vi "MU Calibration Get Analyze Result Log.vi"(8 "error in (no error)":errorcluster, 9 "logLevel":u32, 10 "logDestSize":u64=1024, 11 "analyzeResult":T1) -> (0 "error out (no error)":errorcluster, 2 "logDest":string, 3 "size":u64=1024)   [LabVIEW 2017, in "MU_3SL_interface.lvlib"]
uses:
  MU_3SL_interface.lvlib
  handles/CalibrationAnalyzeResultHandle.ctl
  lib/MU_3SL_interface.dll
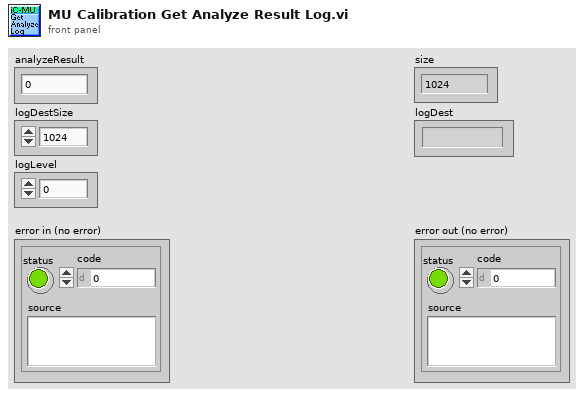
[diagram p1: front panel]
types:
  T1 = typedef "MU_3SL_interface.lvlib/CalibrationAnalyzeResultHandle.ctl" = u64
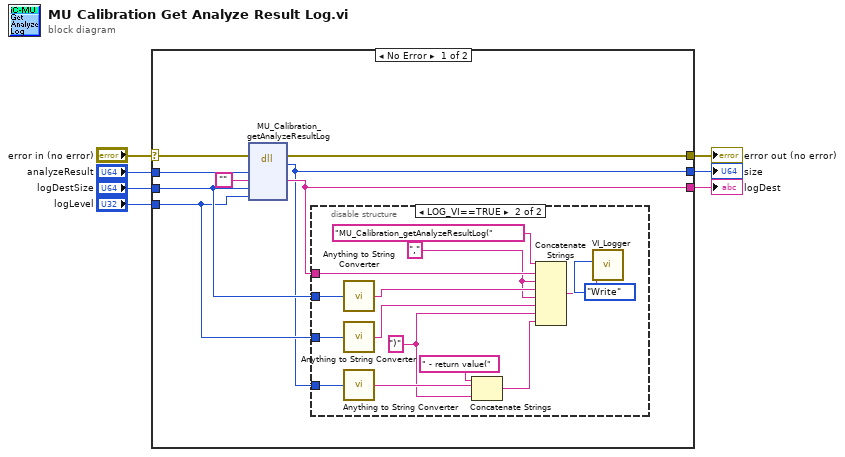
[diagram p0: block diagram]
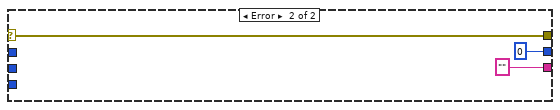
[diagram p3: hidden frame]
diagram:
  n1 = case shown="No Error" "error in (no error)" {
    selector: "error in (no error)" -> [w15 w32]
    tunnel: [w13 w32] -> w7
    tunnel: "analyzeResult" -> [w14 _]
    tunnel: [w9 u64 0 ("size")] -> w1
    tunnel: [w12 "" ("adjustMessage")] -> w4
    tunnel: "logDestSize" -> [w11 _]
    tunnel: "logLevel" -> [w10 _]
    frame No Error {
      n2 = dll-call lib="C:/Users/bes/AppData/Roaming/work/mu_9so/icsubmodules/soft_mu_3sl_master/lv_interface/lib/MU_3SL_interface**.*" fn="MU_Calibration_getAnalyzeResultLog"(error in=w15, "analyzeResultHandle"=w14, "logDest"="", "logDestSize"=w11, "logLevel"=w10) -> (error out=w13:errorcluster, "size"=w9:u64, "logDest"=w12:string)  [unwired: 5 in, 1 out]
      n3 = disable-structure shown="LOG_VI==TRUE" {
        disable-tunnel: w9 -> [_ w25]
        disable-tunnel: w12 -> [_ w23]
        disable-tunnel: w11 -> [_ w22]
        disable-tunnel: w10 -> [_ w21]
        frame condition #0 {
        }
        frame condition #1 (active) {
          w19 = "," ("string")
          w17 = ")" ("string")
          n4 = call "Anything to String Converter.vi"("anything"=w22) -> ("String"=w20:string)
          n5 = call "Anything to String Converter.vi"("anything"=w21) -> ("String"=w18:string)
          n6 = call "Anything to String Converter.vi"("anything"=w25) -> ("String"=w24:string)
          n7 = Concatenate Strings(" - return value(" ("string"), w24, w17) -> (w16:string)
          n8 = Concatenate Strings("MU_Calibration_getAnalyzeResultLog(" ("Info in"), w23, w19, w20, w19, w18, w17, w16) -> (w27:string)
          n9 = call "VI_Logger.vi"("Action (Read)"=enum16{"Write", "Read"}."Write", "Info in"=w27) -> ()  [unwired: 8 in, 2 out]
        }
      }
    }
    frame Error {
    }
  }
  "error out (no error)" <- w7
  "logDest" <- w4
  "size" <- w1
